vi "Measure_SubArray_2(SubVI).vi"(8 "error in (no error)":errorcluster, 9 "FinalPos":dbl, 10 "StartPos":dbl, 11 "InArray":dbl[](array[numeric])) -> (0 "error out":errorcluster, 2 "output cluster":cluster{dbl, dbl, "Numeric Control":dbl, dbl}, 3 "OutSubArray":dbl[](array[numeric]))   [LabVIEW 2014]
doc: "This SubVI calculate SubArray based on start and finish position graph cursors. Then it measure START. MAX and MIN in this SubArray"
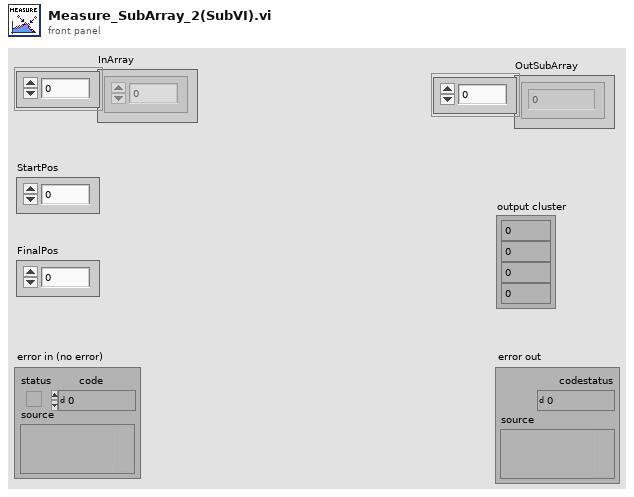
[diagram p1: front panel]
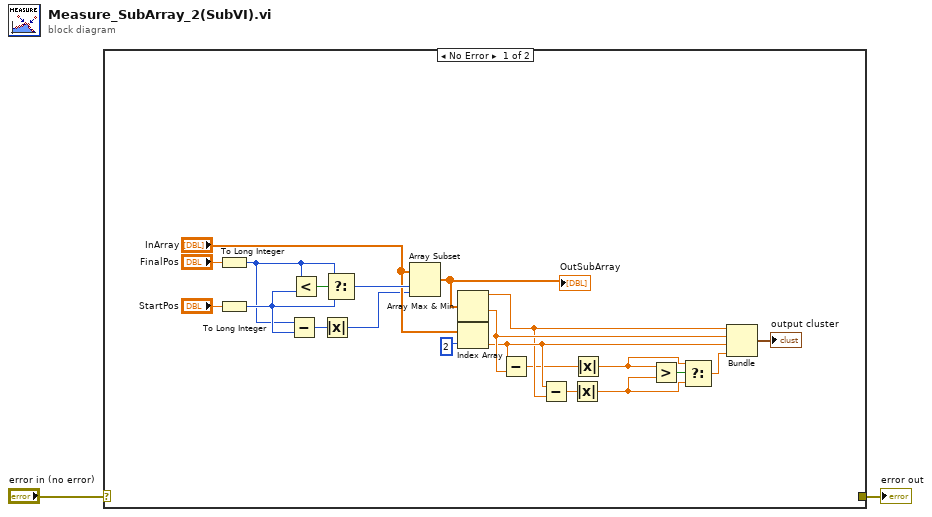
[diagram p0: block diagram]
diagram:
  n1 = case shown="No Error" "error in (no error)" {
    selector: "error in (no error)" -> [_ w24]
    tunnel: [_ w24] -> w1
    frame No Error {
      n2 = To Long Integer(number="FinalPos") -> (32bit integer=w20:i32)
      n3 = To Long Integer(number="StartPos") -> (32bit integer=w21:i32)
      n4 = Subtract(x=w20, y=w21) -> (x-y=w15:i32)
      n5 = Less?(x=w20, y=w21) -> (x < y?=w14:bool)
      n6 = Absolute Value(x=w15) -> (abs(x)=w16:i32)
      n7 = Select(t=w20, s=w14, f=w21) -> (s? t:f=w22:i32)
      n8 = Array Subset(array="InArray", index=w22, length=w16) -> (w23:dbl[])
      "OutSubArray" <- w23
      n9 = Array Max & Min(array=w23) -> (max value=w10:dbl, min value=w12:dbl)  [unwired: 2 out]
      n10 = Index Array(array="InArray", index=2) -> (element=w11:dbl)
      n11 = Subtract(x=w11, y=w12) -> (x-y=w5:dbl)
      n12 = Subtract(x=w11, y=w10) -> (x-y=w6:dbl)
      n13 = Absolute Value(x=w6) -> (abs(x)=w3:dbl)
      n14 = Absolute Value(x=w5) -> (abs(x)=w4:dbl)
      n15 = Greater?(x=w4, y=w3) -> (0:w9:bool)
      n16 = Select(t=w4, s=w9, f=w3) -> (s? t:f=w8:dbl)
      n17 = Bundle(w10, w12, "Numeric Control"=w11, w8) -> (→"output cluster":cluster{dbl, dbl, "Numeric Control":dbl, dbl})  [unwired: 1 in]
    }
    frame Error {
    }
  }
  "error out" <- w1
